vi "Set Tx Generic and Tx UDP Frames from Map.vi"(8 "error in":errorcluster, 10 "payload map":T1 {"value"."Type of Frame" items=["Raw Frame", "UDP/IP Tx Gen", "Tx UDP"]; "value"."Data" format="%.0x"}, 11 "custom device ref":T4 format="%.0x") -> (0 "error out":errorcluster, 3 "custom device ref out":T4 format="%.0x")   [LabVIEW 2020, in "AIM ARINC 664 Scripting.lvlib"]
uses:
  AIM ARINC 664 Scripting.lvlib
  <vilib>/NI VeriStand/Custom Device API/Custom Device Item Ref.ctl
  Frame Configuration/controls/Payload Map.ctl
  Frame Configuration/controls/Payload Record Type.ctl
  Frame Configuration/controls/Type of Payload.ctl
  40cee884-5832-4c51-a00e-06261b7629d9.vi
  0f87c89b-799f-4781-a9f9-0be7cbb0cd91.vi
  Constants.vi
  <vilib>/NI VeriStand/Custom Device Tools/Custom Device Utility Library/NI VeriStand - Search for All Items by GUID.vi
  <vilib>/NI VeriStand/Custom Device API/Get Item Property (String).vi
  <vilib>/NI VeriStand/Custom Device API/Set Item Property (Variant).vi
  <vilib>/Comparison/Less/Less Functor/Less Functor.lvclass
  <vilib>/NI VeriStand/Custom Device Tools/Custom Device Utility Library/Custom Device Utility Library.lvlib
  <vilib>/NI VeriStand/Custom Device API/Custom Device API.lvlib
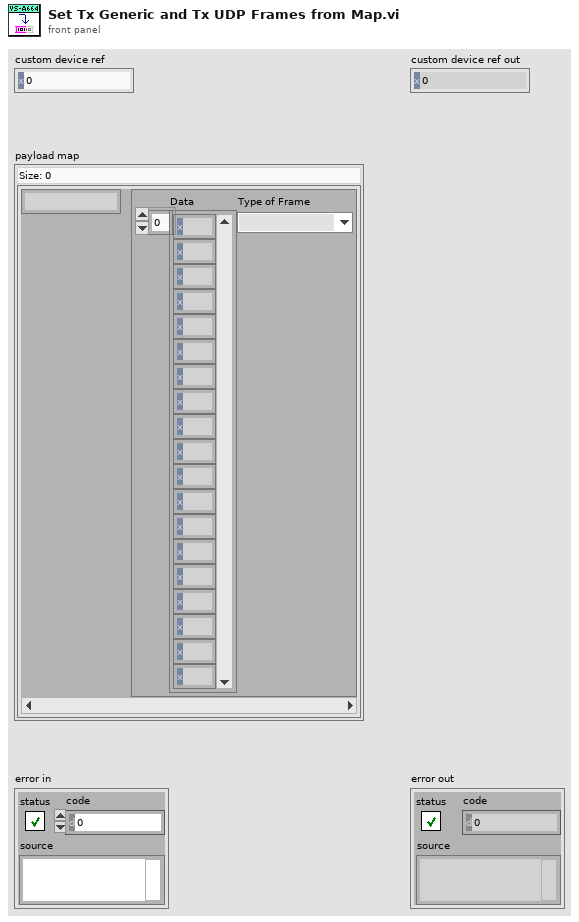
[diagram p1: front panel]
types:
  T1 = typedef "Payload Map.ctl" = map{string, T2}
  T2 = typedef "Payload Record Type.ctl" = cluster{"Data":u8[], "Type of Frame":T3}
  T3 = typedef "Type of Payload.ctl" = u16
  T4 = typedef "Custom Device API.lvlib/Custom Device Item Ref.ctl" = u64
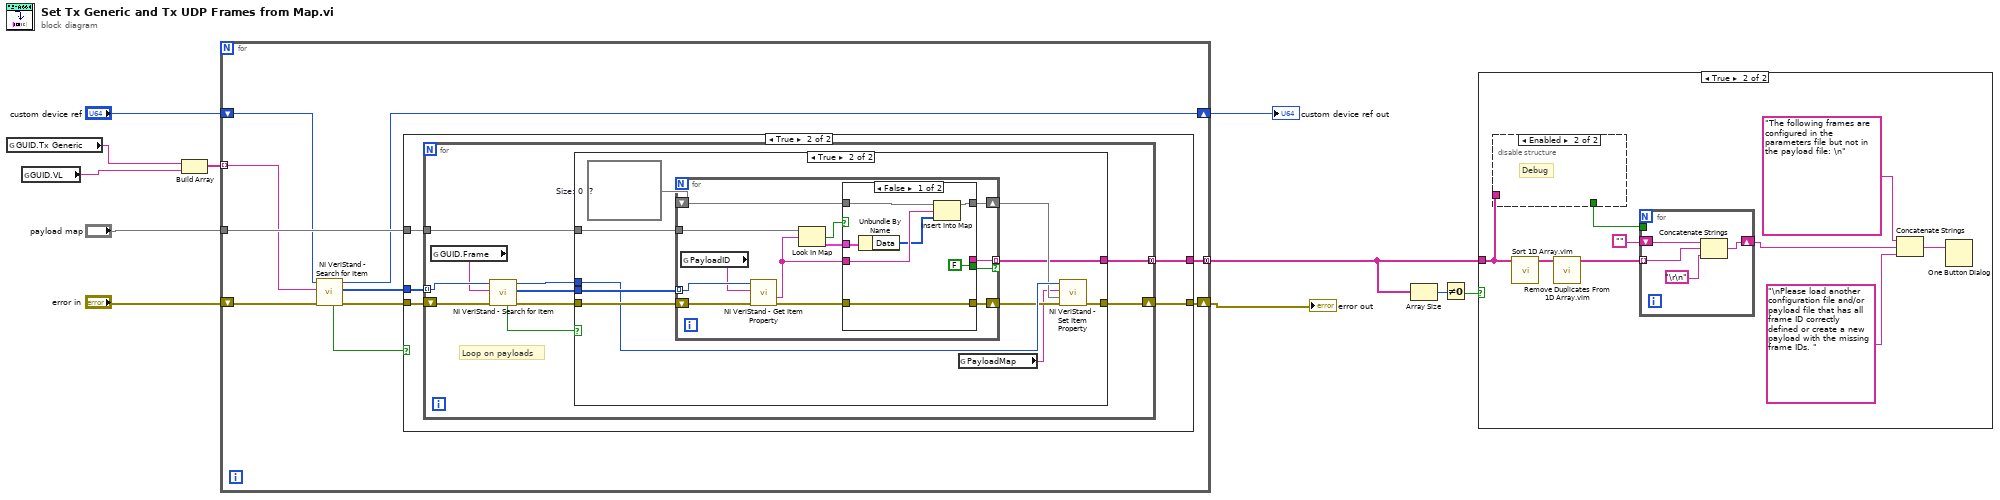
[diagram p0: block diagram]
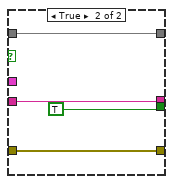
[diagram p4: hidden frame]
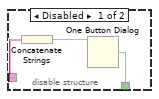
[diagram p6: hidden frame]
diagram:
  n1 = global read "Constants.vi" "GUID.Tx Generic"() -> (w2:string)
  n2 = global read "Constants.vi" "GUID.VL"() -> (w1:string)
  n3 = Build Array(w2, w1) -> (w3:string[])
  n4 = for {
    tunnel: "payload map" -> [w20]
    tunnel: [w16] -> w6 mode=concatenating
    shift-right: [w21] -> w11
    shift-left: "error in" -> [w19]
    shift-right: [w17] -> w7
    shift-left: "custom device ref" -> [w18]
    tunnel: w3 -> [w12] mode=indexing
    n5 = call-poly <vilib>:"NI VeriStand - Search for Item.vi"("error in"=w19, "Item GUID"=w12, "Section Ref in"=w18) -> ("error out"=w14:errorcluster, "Item Refs"=w13:T4[], "Section Ref out"=w17:T4, "Found"=w15:bool)  [unwired: 5 in]
    n6 = case shown="True" w15 {
      tunnel: w14 -> [w22 w27]
      tunnel: w13 -> [_ w26]
      tunnel: [w22 w25] -> w21
      tunnel: w20 -> [_ w24]
      tunnel: [_ w23] -> w16
      frame False {
      }
      frame True {
        n7 = for {
          shift-right: [w33] -> w25
          shift-left: w27 -> [w37]
          tunnel: w26 -> [w30] mode=indexing
          tunnel: w24 -> [w32]
          tunnel: [w31] -> w23 mode=concatenating
          # "Loop on payloads"
          n8 = global read "Constants.vi" "GUID.Frame"() -> (w29:string)
          n9 = call-poly <vilib>:"NI VeriStand - Search for Item.vi"("error in"=w37, "Item GUID"=w29, "Section Ref in"=w30) -> ("error out"=w34:errorcluster, "Item Refs"=w35:T4[], "Section Ref out"=w28:T4, "Found"=w36:bool)  [unwired: 5 in]
          n10 = case shown="True" w36 {
            tunnel: w35 -> [_ w47]
            tunnel: w34 -> [w38 w48]
            tunnel: [w38 w42] -> w33
            tunnel: w32 -> [_ w46]
            tunnel: w28 -> [_ w44]
            tunnel: [_ w40] -> w31
            frame False {
            }
            frame True {
              w45 = map{string, u8[]} {}  # Size: 0
              n11 = for {
                shift-right: [w55] -> w43
                shift-left: w48 -> [w61]
                tunnel: w47 -> [w60] mode=indexing
                tunnel: w46 -> [w58]
                shift-right: [w53] -> w41
                shift-left: w45 -> [w52]
                tunnel: [w56] -> w40 mode=indexing if=w54
                n12 = global read "Constants.vi" "PayloadID"() -> (w59:string)
                n13 = call-poly <vilib>:"NI VeriStand - Get Item Property.vi"("error in (no error)"=w61, "Property Name"=w59, "Item Ref in"=w60) -> ("error out"=w57:errorcluster, "Value"=w50:string)  [unwired: 5 in, 2 out]
                n14 = Look In Map(map=w58, key=w50) -> (key not found?=w49:bool, value=w51:T2)  [unwired: 1 in]
                n15 = case shown="False" w49 {
                  tunnel: w57 -> [w63 w71]
                  tunnel: [_ w72] -> w56
                  tunnel: w50 -> [w65 w72]
                  tunnel: [w63 w71] -> w55
                  tunnel: [FALSE TRUE] -> w54
                  tunnel: [w67 w69] -> w53
                  tunnel: w52 -> [w68 w69]
                  tunnel: w51 -> [w66 _]
                  frame False {
                    n16 = Unbundle By Name(w66) -> ("Data"=w62:u8[])
                    n17 = Insert Into Map(map in=w68, key=w65, value=w62) -> (map out=w67:map{string, u8[]})  [unwired: 2 out]
                  }
                  frame True {
                  }
                }
              }
              n18 = global read "Constants.vi" "PayloadMap"() -> (w39:string)
              n19 = call-poly <vilib>:"NI VeriStand - Set Item Property.vi"("error in (no error)"=w43, "Value"=w41, "Property Name"=w39, "Item Ref in"=w44) -> ("error out"=w42:errorcluster)  [unwired: 5 in, 2 out]
            }
          }
        }
      }
    }
  }
  "error out" <- w11
  "custom device ref out" <- w7
  n20 = Array Size(array=w6) -> (size(s)=w5:i32)
  n21 = Not Equal To 0?(x=w5) -> (x != 0?=w4:bool)
  n22 = case shown="True" w4 {
    tunnel: w6 -> [_ w74]
    frame False {
    }
    frame True {
      n23 = disable-structure shown="Enabled" {
        disable-tunnel: w74 -> [w83 _]
        disable-tunnel: [w82 _] -> w73
        frame Disabled {
          n24 = Concatenate Strings(w83) -> (w84:string)
          n25 = One Button Dialog(message=w84) -> (true=w82:bool)  [unwired: 1 in]
        }
        frame Enabled {
          # "Debug"
        }
      }
      n26 = call "Sort 1D Array.vim"("unsorted array"=w74) -> ("sorted array"=w78:string[])  [unwired: 10 in]
      n27 = call "Remove Duplicates From 1D Array.vim"("array"=w78) -> ("array with duplicates removed"=w77:string[])  [unwired: 10 in]
      n28 = for {
        tunnel: w77 -> [w88] mode=indexing
        shift-right: [w85] -> w75
        shift-left: "" -> [w86]
        tunnel: w73 -> [_]
        n29 = Concatenate Strings(w86, w88, "\r\n") -> (w85:string)
      }
      n30 = Concatenate Strings("The following frames are configured in the parameters file but not in the payload file: \n" ("message"), w75, "\nPlease load another configuration file and/or payload file that has all frame ID correctly defined or create a new payload with the missing frame IDs. " ("message")) -> (w80:string)
      n31 = One Button Dialog(message=w80) -> ()  [unwired: 1 in, 1 out]
    }
  }
